vi "P9685Servo-Motor_Test.vi"() -> ()   [LabVIEW 2019]
panel:
  in  "角度4":dbl(knob) scale=0.0..180.0
  in  "角度3":dbl(knob) scale=0.0..180.0
  in  "PWM腳位 4":T1(ring)=enum."LED/PWM03"
  in  "PWM腳位 3":T1(ring)=enum."LED/PWM02"
  in  "PWM腳位 2":T1(ring)=enum."LED/PWM01"
  in  "PWM腳位":T1(ring)
  in  "Error In":errorcluster
  out "error out":errorcluster
  in  "角度2":dbl(knob) scale=0.0..180.0
  in  "角度":dbl(knob) scale=0.0..180.0
  in  "Stop":bool
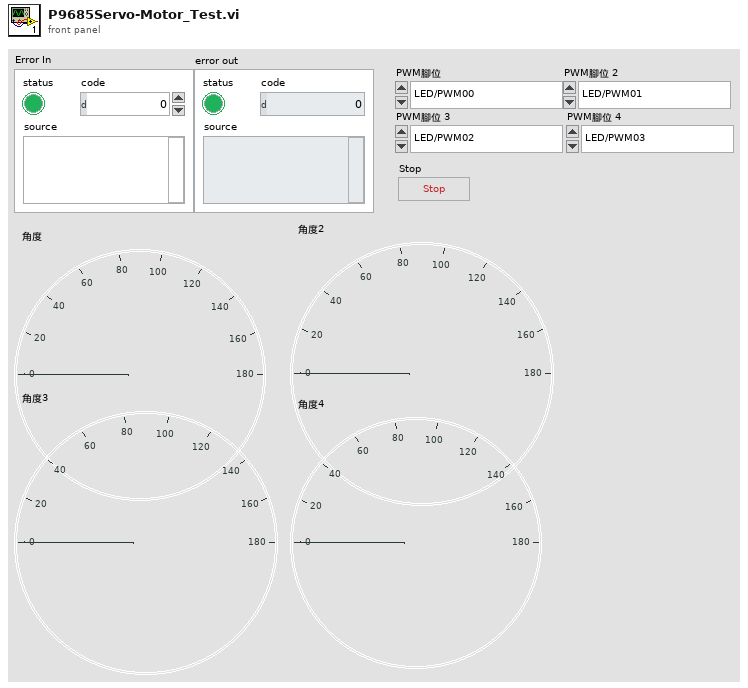
[diagram p1: front panel]
types:
  T1 = enum16{"LED/PWM00", "LED/PWM01", "LED/PWM02", "LED/PWM03", "LED/PWM04", "LED/PWM05", "LED/PWM06", "LED/PWM07", "LED/PWM08", "LED/PWM09", "LED/PWM10", "LED/PWM11", "LED/PWM12", "LED/PWM13", "LED/PWM14", "LED/PWM15"}
  T2 = typedef "I2C.lvlib/I2C Reference.ctl" = cluster{"myRIO Reference":T3, "I2C Channels Enum":T7, "I2C Configuration":T8}
  T3 = typedef "myRIO Generic Hardware Reference.ctl" = cluster{"myRIO Model":T4, "myRIO Hardware Reference":T5}
  T4 = typedef "Hardware Version Enum.ctl" = enum16{"Unknown", "myRIO-1900", "myRIO-1950", "roboRIO", "NI ELVIS RIO CM", "ELVIS III"}
  T5 = typedef "myRIO v1.0 Reference.ctl" = cluster{"Generic FPGA Reference":T6, "Allow multiple opens":bool}
  T6 = typedef "Generic FPGA Reference.ctl" = refnum<k20>
  T7 = typedef "I2C Channels Enum.ctl" = enum16{"Not Connected", "A/I2C", "B/I2C", "I2C/I2C"}
  T8 = typedef "I2C.lvlib/I2C Configuration.ctl" = cluster{"I2C Transfer Rate":T9}
  T9 = typedef "I2C.lvlib/I2C Transfer Rate.ctl" = enum16{"Standard mode (100 kbps)", "Fast mode (400 kbps)"}
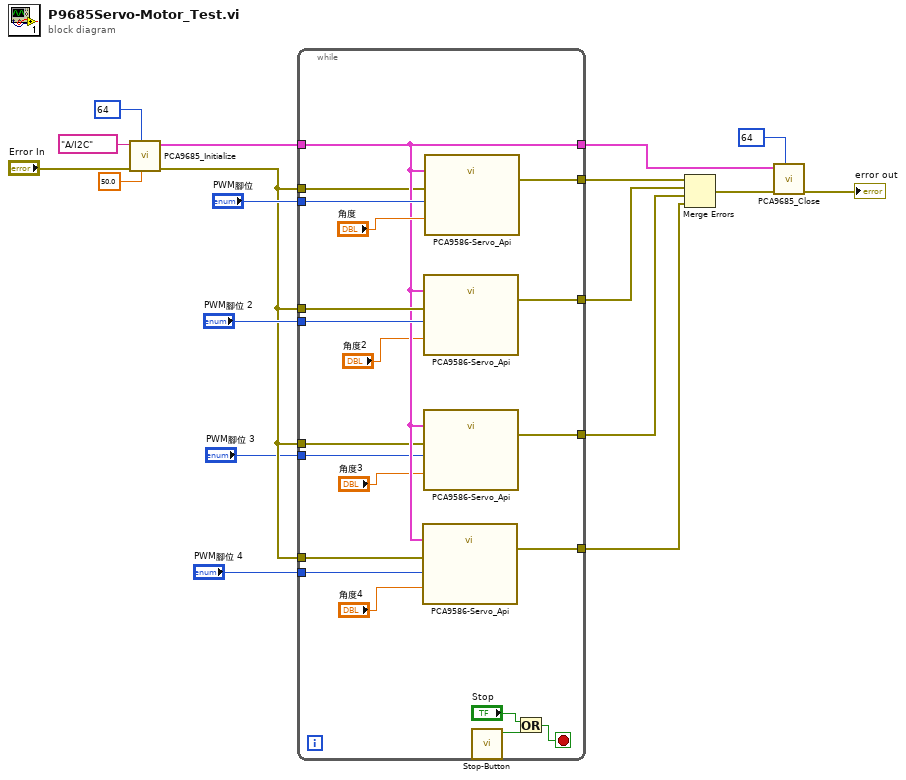
[diagram p0: block diagram]
diagram:
  n1 = call "PCA9685_Initialize.vi"("PWM頻率(50Hz)"=50.0, "驅動板位址(0x40)"=u8 64, "Error In"="Error In", "I2C腳位"=tag "A/I2C") -> ("Error Out"=w3:errorcluster, "I2C Ref Out"=w9:T2)  [unwired: 6 in]
  n2 = while {
    tunnel: w3 -> [w26]
    tunnel: w3 -> [w35]
    tunnel: "PWM腳位" -> [w33]
    tunnel: "PWM腳位 2" -> [w32]
    tunnel: w9 -> [w31]
    tunnel: [w31] -> w8
    tunnel: [w30] -> w7
    tunnel: [w29] -> w6
    tunnel: [w28] -> w5
    tunnel: [w27] -> w4
    tunnel: w3 -> [w25]
    tunnel: w3 -> [w24]
    tunnel: "PWM腳位 3" -> [w23]
    tunnel: "PWM腳位 4" -> [w22]
    stop <- w36 stop-if-true
    n3 = call "PCA9586-Servo_Api.vi"("Error In"=w24, "角度"="角度4", "I2C Ref In"=w31, "PWM腳位"=w22) -> ("Error Out"=w27:errorcluster)  [unwired: 7 in]
    n4 = call "PCA9586-Servo_Api.vi"("Error In"=w35, "角度"="角度2", "I2C Ref In"=w31, "PWM腳位"=w32) -> ("Error Out"=w29:errorcluster)  [unwired: 7 in]
    n5 = call "PCA9586-Servo_Api.vi"("Error In"=w25, "角度"="角度3", "I2C Ref In"=w31, "PWM腳位"=w23) -> ("Error Out"=w28:errorcluster)  [unwired: 7 in]
    n6 = call "PCA9586-Servo_Api.vi"("Error In"=w26, "角度"="角度", "I2C Ref In"=w31, "PWM腳位"=w33) -> ("Error Out"=w30:errorcluster)  [unwired: 7 in]
    n7 = call "Stop-Button.vi"() -> ("顯示按下?"=w38:bool)  [unwired: 10 in, 1 out]
    n8 = Or(x="Stop", y=w38) -> (x .or. y?=w36:bool)
  }
  n9 = Merge Errors(w7, w6, w5, w4) -> (w16:errorcluster)
  n10 = call "PCA9685_Close.vi"("驅動板位址(0x40)"=u8 64, "Error In"=w16, "I2C Ref In"=w8) -> ("Error Out"=→"error out":errorcluster)  [unwired: 8 in]
